vi "Run Test.vi"(8 "error in (no error)":errorcluster, 11 "Test Template in":refnum<class "Rocom Connect.lvclass">) -> (0 "error out":errorcluster, 1 "Fail Codes":string[](array[string]), 2 "Tests Passed":bool[](array[boolean]), 3 "Test Template out":refnum<class "Rocom Connect.lvclass">)   [LabVIEW 2015, in "Rocom Connect.lvclass"]
uses:
  Rocom Connect.lvclass
  Test Class/Test Class.lvclass
  Classes/Application/Class/Application.lvclass
  Rocom Tests/Rocom Tests.lvclass
  Classes/Manufacturing Test/Class/SC Manufacturing Test.lvclass
  <vilib>/Cree, Inc/Cree Test Framework/Classes/Base Objects/Base Class/Base Class/Base Class.lvclass
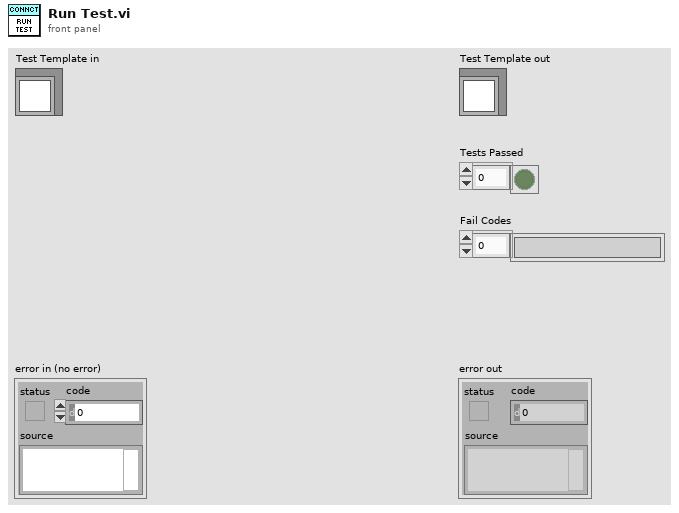
[diagram p1: front panel]
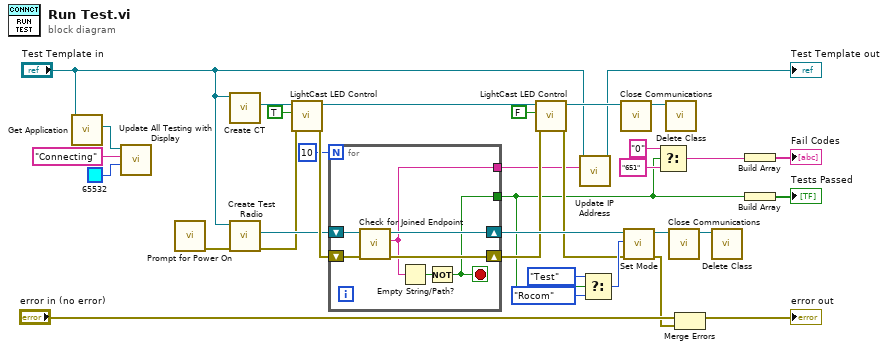
[diagram p0: block diagram]
diagram:
  n1 = call "Get Application.vi"("Test Class in"="Test Template in") -> ("Application.lvlib:Application.lvclass"=w32:refnum<class "Application.lvclass">)  [unwired: 9 in, 1 out]
  n2 = call "Update All Testing with Display.vi"("BG Color"=u32 65532, "Message ('')"="Connecting", "Application in"=w32) -> ()  [unwired: 7 in, 2 out]
  n3 = call "Prompt for Power On.vi"() -> ("Error out"=w1:errorcluster)  [unwired: 10 in, 1 out]
  n4 = call "Create CT.vi"("Rocom Tests in"="Test Template in") -> ("Test Radio"=w20:refnum<class "SC Manufacturing Test.lvclass">)  [unwired: 8 in, 2 out]
  n5 = call "Create Test Radio.vi"("error in (no error)"=w1, "Rocom Tests in"="Test Template in") -> ("error out"=w5:errorcluster, "Test Radio"=w19:refnum<class "SC Manufacturing Test.lvclass">)  [unwired: 7 in, 1 out]
  n6 = call "LightCast LED Control.vi"("error in (no error)"=w5, "On/Off (Off)"=TRUE, "Acrobat Template in"=w20) -> ("error out"=w29:errorcluster, "Acrobat Template out"=w30:refnum<class "SC Manufacturing Test.lvclass">)  [unwired: 7 in]
  n7 = for {
    N: 10 -> [_]
    shift-right: [w39] -> w31
    shift-left: w19 -> [w41]
    shift-right: [w38] -> w21
    shift-left: w29 -> [w40]
    tunnel: [w36] -> w3
    tunnel: [w35] -> w10
    stop <- w36 stop-if-true
    n8 = call "Check for Joined Endpoint.vi"("error in (no error)"=w40, "Acrobat Template in"=w41) -> ("error out"=w38:errorcluster, "IPv6 Address"=w35:string, "Acrobat Template out"=w39:refnum<class "SC Manufacturing Test.lvclass">)  [unwired: 7 in]
    n9 = Empty String/Path?(string/path=w35) -> (empty?=w37:bool)
    n10 = Not(x=w37) -> (.not. x?=w36:bool)
  }
  n11 = call "LightCast LED Control.vi"("error in (no error)"=w21, "On/Off (Off)"=FALSE, "Acrobat Template in"=w30) -> ("error out"=w22:errorcluster, "Acrobat Template out"=w9:refnum<class "SC Manufacturing Test.lvclass">)  [unwired: 7 in]
  n12 = call "Update IP Address.vi"("IP Address"=w10, "Rocom Tests in"="Test Template in") -> ("Rocom Tests out"=→"Test Template out":refnum<class "Rocom Connect.lvclass">)  [unwired: 8 in, 1 out]
  n13 = Select(t=enum16{"Normal", "Test", "Rocom"}."Test" ("Mode"), s=w3, f=enum16{"Normal", "Test", "Rocom"}."Rocom" ("Mode")) -> (s? t:f=w28:enum16{"Normal", "Test", "Rocom"})
  n14 = call "Close Communications.vi"("Acrobat Template in"=w9) -> ("Acrobat Template out"=w8:refnum<class "SC Manufacturing Test.lvclass">)  [unwired: 9 in, 1 out]
  n15 = call "Set Mode.vi"("error in (no error)"=w22, "Mode"=w28, "Acrobat Template in"=w31) -> ("error out"=w16:errorcluster, "Acrobat Template out"=w7:refnum<class "SC Manufacturing Test.lvclass">)  [unwired: 7 in]
  n16 = Select(t="0" ("Message ('')"), s=w3, f="651" ("Message ('')")) -> (s? t:f=w12:string)
  n17 = call <vilib>:"Delete Class.vi"("Base Class in"=w8) -> ()  [unwired: 9 in, 2 out]
  n18 = call "Close Communications.vi"("Acrobat Template in"=w7) -> ("Acrobat Template out"=w6:refnum<class "SC Manufacturing Test.lvclass">)  [unwired: 9 in, 1 out]
  n19 = Merge Errors("error in (no error)", w16) -> (→"error out":errorcluster)
  n20 = call <vilib>:"Delete Class.vi"("Base Class in"=w6) -> ()  [unwired: 9 in, 2 out]
  n21 = Build Array(w12) -> (→"Fail Codes":string[])
  n22 = Build Array(w3) -> (→"Tests Passed":bool[])
